vi "Obtain Queues.vi"() -> (0 "error out":errorcluster, 3 "msg cluster":T1)   [LabVIEW 2020]
uses:
  Messaging Cluster.ctl
  Hardware/Sensors/Cameras/Camera.lvclass
  Hardware/Sensors/Force Sensors/Force Sensor.lvclass
  Hardware/Actuators/Servos/Servo.lvclass
  Hardware/Actuators/Switches/Switch.lvclass
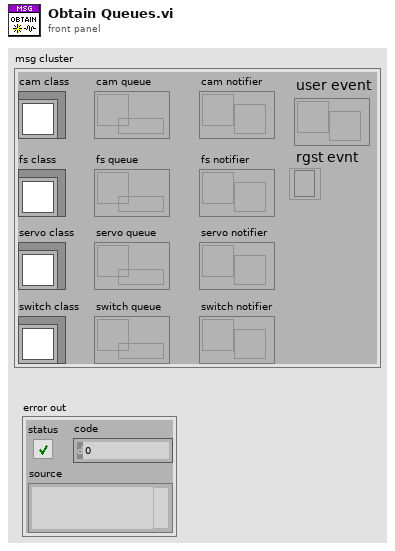
[diagram p1: front panel]
types:
  T1 = typedef "Messaging Cluster.ctl" = cluster{"cam queue":refnum<queue>, "fs queue":refnum<queue>, "servo queue":refnum<queue>, "switch queue":refnum<queue>, "cam class":refnum<class "Camera.lvclass">, "fs class":refnum<class "Force Sensor.lvclass">, "servo class":refnum<class "Servo.lvclass">, "switch class":refnum<class "Switch.lvclass">, "switch notifier":refnum<notifier>, "servo notifier":refnum<notifier>, "fs notifier":refnum<notifier>, "cam notifier":refnum<notifier>, "rgst evnt":refnum<event-registration>, "user event":refnum<user-event>}
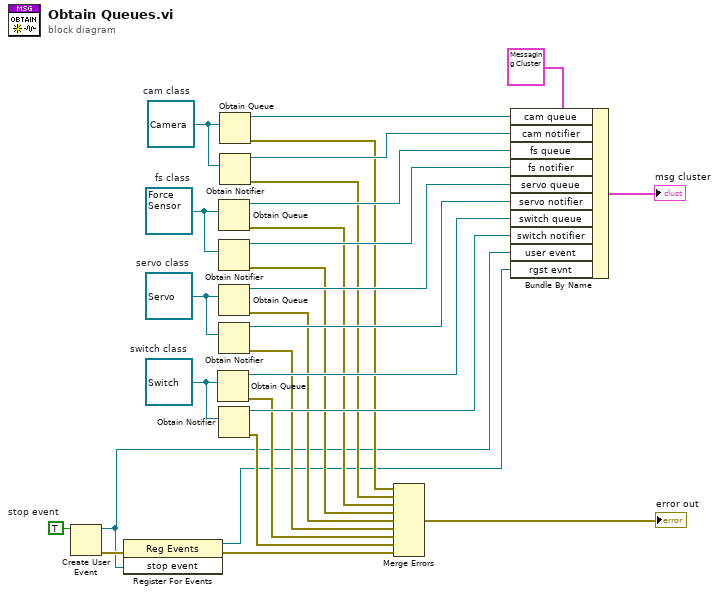
[diagram p0: block diagram]
diagram:
  w4 = TRUE  # stop event
  w21 = refnum<class "Force Sensor.lvclass"> refnum  # fs class
  w22 = refnum<class "Camera.lvclass"> refnum  # cam class
  w23 = refnum<class "Servo.lvclass"> refnum  # servo class
  w24 = refnum<class "Switch.lvclass"> refnum  # switch class
  n1 = Create User Event(user event datatype=w4) -> (user event=w2:refnum<user-event>, error out=w5:errorcluster)  [unwired: 1 in]
  n2 = register-events(error in=w5, w2) -> (reference out=w1:refnum<event-registration>, error out=w3:errorcluster)  [unwired: 1 in]
  n3 = Obtain Queue(element data type=w24) -> (queue out=w15:refnum<queue>, error out=w12:errorcluster)  [unwired: 4 in, 1 out]
  n4 = Obtain Queue(element data type=w21) -> (queue out=w19:refnum<queue>, error out=w8:errorcluster)  [unwired: 4 in, 1 out]
  n5 = Obtain Notifier(notification data type=w21) -> (notifier out=w18:refnum<notifier>, error out=w9:errorcluster)  [unwired: 3 in, 1 out]
  n6 = Obtain Queue(element data type=w23) -> (queue out=w17:refnum<queue>, error out=w10:errorcluster)  [unwired: 4 in, 1 out]
  n7 = Obtain Notifier(notification data type=w23) -> (notifier out=w16:refnum<notifier>, error out=w11:errorcluster)  [unwired: 3 in, 1 out]
  n8 = Obtain Notifier(notification data type=w24) -> (notifier out=w14:refnum<notifier>, error out=w13:errorcluster)  [unwired: 3 in, 1 out]
  n9 = Obtain Queue(element data type=w22) -> (queue out=w27:refnum<queue>, error out=w6:errorcluster)  [unwired: 4 in, 1 out]
  n10 = Obtain Notifier(notification data type=w22) -> (notifier out=w20:refnum<notifier>, error out=w7:errorcluster)  [unwired: 3 in, 1 out]
  n11 = Merge Errors(w6, w7, w8, w9, w10, w11, w12, w13, w3) -> (→"error out":errorcluster)
  n12 = Bundle By Name(cluster=T1 {"cam queue"=refnum, "fs queue"=refnum, "servo queue"=refnum, "switch queue"=refnum, "cam class"=refnum, "fs class"=refnum, "servo class"=refnum, "switch class"=refnum, "switch notifier"=refnum, "servo notifier"=refnum, "fs notifier"=refnum, "cam notifier"=refnum, "rgst evnt"=refnum, "user event"=refnum}, "cam queue"=w27, "cam notifier"=w20, "fs queue"=w19, "fs notifier"=w18, "servo queue"=w17, "servo notifier"=w16, "switch queue"=w15, "switch notifier"=w14, "user event"=w2, "rgst evnt"=w1) -> (→"msg cluster":T1)
